vi "Read Database.vi"(8 "error in (no error)":errorcluster, 11 "Table Configuration Basic DB in":refnum<class "Table Configuration Basic DB.lvclass">) -> (0 "error out":errorcluster, 2 "Database":refnum<class "Database Interface.lvclass">, 3 "Table Configuration Basic DB out":refnum<class "Table Configuration Basic DB.lvclass">)   [LabVIEW 2020]
uses:
  Table Configuration Basic DB.lvclass
  C:/Users/User/Desktop/Raman Program/Database OOP/source/Database OOP/Table Configuration/Table Configuration.lvclass
  C:/Users/User/Desktop/Raman Program/Database OOP/source/Database OOP/Table Configuration Interface/Table Configuration Interface.lvclass
  C:/Users/User/Desktop/Raman Program/Database OOP/source/Database OOP/Table Configuration Basic DB/Table Configuration Basic DB.lvclass
  Database Interfaces/Database Interface Class/Database Interface.lvclass
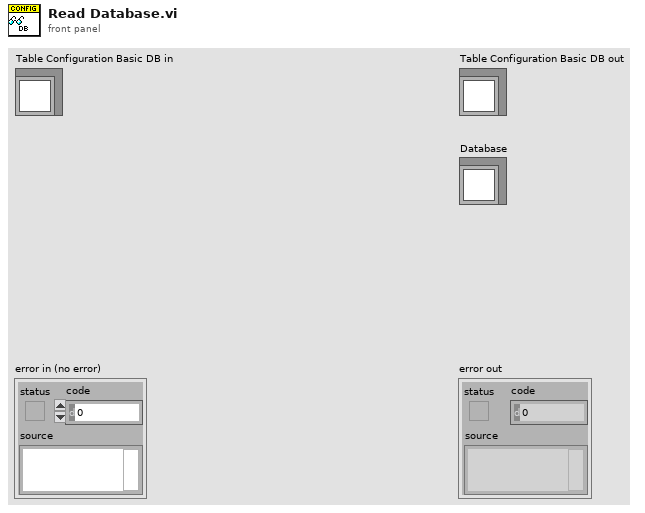
[diagram p1: front panel]
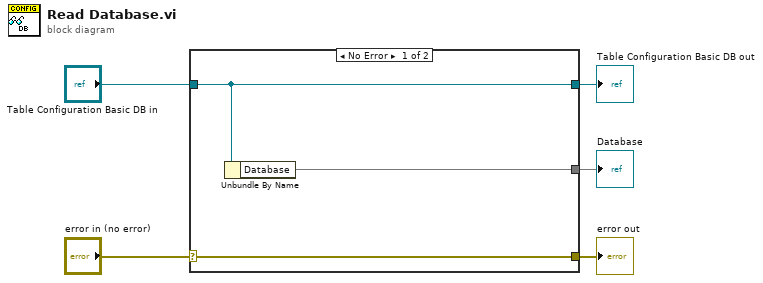
[diagram p0: block diagram]
diagram:
  n1 = case shown="No Error" "error in (no error)" {
    selector: "error in (no error)" -> [w8 w9]
    tunnel: [w8 w9] -> w4
    tunnel: [w7 w10] -> w2
    tunnel: "Table Configuration Basic DB in" -> [w7 w10]
    tunnel: [w6 _] -> w1
    frame No Error {
      n2 = Unbundle By Name(w7) -> ("Database"=w6)
    }
    frame Error {
    }
  }
  "error out" <- w4
  "Table Configuration Basic DB out" <- w2
  "Database" <- w1
